vi "Get Auxiliary Amplifier.vi"(8 "error in (no error)":errorcluster, 11 "VISA resource name":refnum<visa-resource-name>) -> (0 "error out":errorcluster, 1 "Current Boost":i32, 2 "Voltage Boost":i32, 3 "VISA resource name out":refnum<visa-resource-name>)   [LabVIEW 2013, in "Fluke 5XXX Series Multicalibrators.lvlib"]
doc: "This VI returns the model numbers of auxiliary amplifiers selected for voltage and current boost.\n\nNote:\n\nThis VI is available only for instrument models 5700A and 5720A."
uses:
  Fluke 5XXX Series Multicalibrators.lvlib
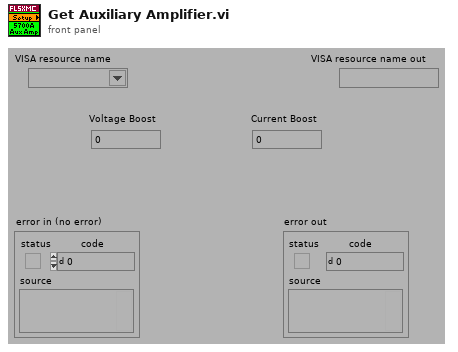
[diagram p1: front panel]
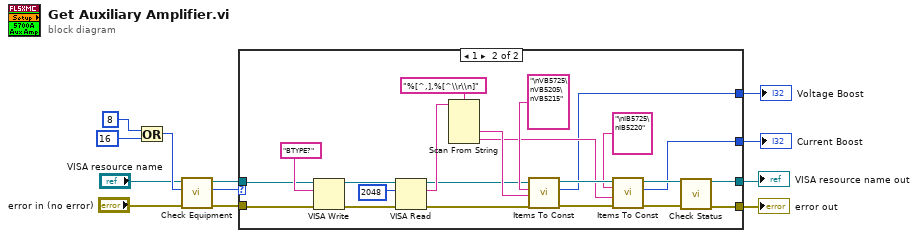
[diagram p0: block diagram]
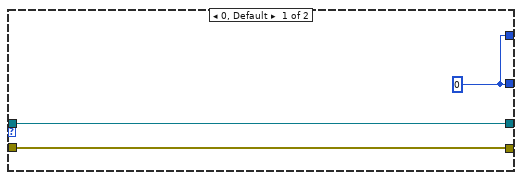
[diagram p2: hidden frame]
diagram:
  n1 = Or(x=8 ("Numeric"), y=16 ("Numeric")) -> (x .or. y?=w7:i32)
  n2 = call "Check Equipment.vi"("error in (no error)"="error in (no error)", "Bit Mask"=w7, "VISA resource name"="VISA resource name") -> ("error out"=w12:errorcluster, "Present?"=w11:u32, "VISA resource name out"=w10:refnum<visa-resource-name>)  [unwired: 6 in]
  n3 = case shown="1" w11 {
    tunnel: [w15 w31] -> w4
    tunnel: [w14 w30] -> w3
    tunnel: w12 -> [w15 w33]
    tunnel: w10 -> [w14 w32]
    tunnel: [w13 w17] -> w2
    tunnel: [w13 w16] -> w1
    frame 0, Default {
      w13 = 0
    }
    frame 1 {
      n4 = VISA Write(VISA resource name=w32, write buffer="BTYPE?", error in (no error)=w33) -> (VISA resource name out=w36:refnum<visa-resource-name>, error out=w35:errorcluster)  [unwired: 1 out]
      n5 = VISA Read(VISA resource name=w36, byte count=u32 2048 ("byte count (0)"), error in (no error)=w35) -> (VISA resource name out=w20:refnum<visa-resource-name>, read buffer=w28:string, error out=w23:errorcluster)  [unwired: 1 out]
      n6 = Scan From String(format string="%[^,],%[^\\r\\n]", input string=w28) -> (output 1=w22:string, output 2=w18:string)  [unwired: 4 in, 3 out]
      n7 = call "Items To Const.vi"("error in (no error)"=w23, "String Item"=w22, "Multi-Line String"="\nVB5725\nVB5205\nVB5215", "VISA resource name"=w20) -> ("error out"=w24:errorcluster, "Index"=w17:i32, "VISA resource name out"=w27:refnum<visa-resource-name>)  [unwired: 5 in]
      n8 = call "Items To Const.vi"("error in (no error)"=w24, "String Item"=w18, "Multi-Line String"="\nIB5725\nIB5220", "VISA resource name"=w27) -> ("error out"=w25:errorcluster, "Index"=w16:i32, "VISA resource name out"=w26:refnum<visa-resource-name>)  [unwired: 5 in]
      n9 = call "Check Status.vi"("VISA resource name"=w26, "error in (no error)"=w25) -> ("VISA resource name out"=w30:refnum<visa-resource-name>, "error out"=w31:errorcluster)  [unwired: 12 in]
    }
  }
  "Voltage Boost" <- w2
  "Current Boost" <- w1
  "VISA resource name out" <- w3
  "error out" <- w4
